vi "Camera.vi"(11 "error in (no error)":errorcluster) -> (0 "Time Out (ms) 2":u8, 1 "Camera 2":bool, 2 "Feature listout":u16, 3 "Out":bool)   [LabVIEW 2015]
uses:
  Control Button/Exit.ctl
  Control PB/Next_.ctl
panel:
  in  "Feature list":u16(ring) items=["LCD/TFT & Dail Check Camera", "CAM2", "CAM3"]
  in  "Camera":bool
  in  "Time Out (ms)":u8
  in  "Next":T1
  in  "Exit":T2
  # "Add Feature List"
  # "CAM1"
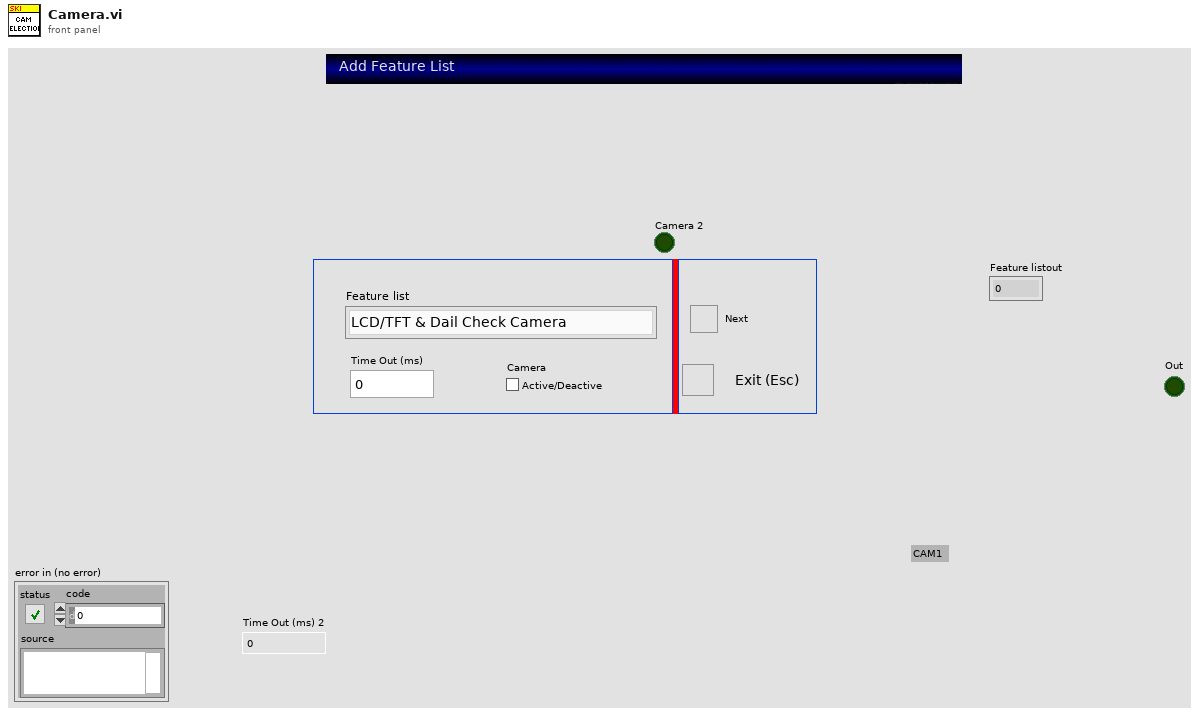
[diagram p1: front panel]
types:
  T1 = typedef "Next_.ctl" = bool
  T2 = typedef "Exit.ctl" = bool
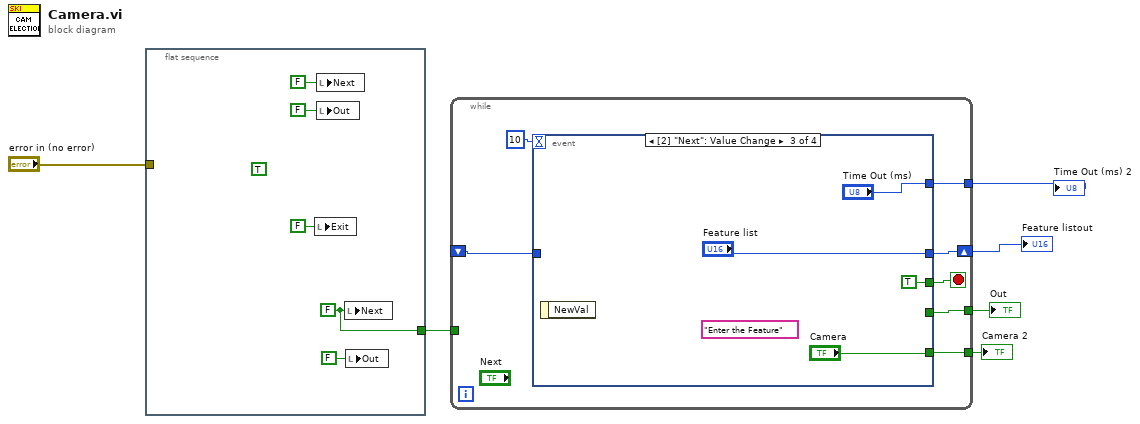
[diagram p0: block diagram]
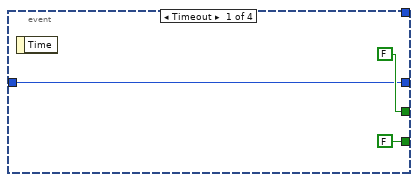
[diagram p2: hidden frame]
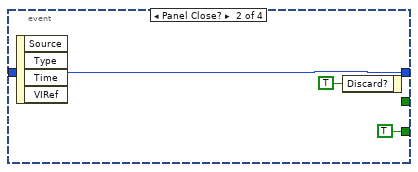
[diagram p3: hidden frame]
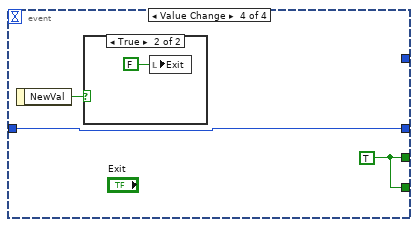
[diagram p4: hidden frame]
diagram:
  n1 = flat-sequence {
    tunnel: [w8] -> w5
    tunnel: "error in (no error)" -> [_]
    frame #0 {
      w8 = T1 FALSE ("Next")
      (unwired) TRUE ("Key Focus")
      n2 = local write "Exit"(FALSE ("Exit")) -> ()
      n3 = local write "Next"(T1 FALSE ("Next")) -> ()
      n4 = local write "Out"(FALSE ("Out")) -> ()
      n5 = local write "Next"(w8) -> ()
      n6 = local write "Out"(FALSE ("Out")) -> ()
    }
  }
  n7 = while {
    tunnel: [w16] -> w6
    tunnel: w5 -> [_]
    shift-right: [w17] -> w1
    shift-left: _ -> [w14]
    tunnel: [w13] -> w4
    tunnel: [w12] -> w3
    stop <- w18 stop-if-true
    n8 = event shown="[2] \"Next\": Value Change" {
      selector: _ -> [_ _ _ _]
      dyn-events: _ -> [_ _ _ _]
      timeout: 10 -> [_ _ _ _]
      tunnel: [FALSE _ TRUE w29] -> w18
      tunnel: [w19 w22 "Feature list" w30] -> w17
      tunnel: [T1 FALSE ("NewVal") T1 TRUE ("NewVal") _ w29] -> w16
      tunnel: w14 -> [w19 w22 _ w30]
      tunnel: [_ _ "Time Out (ms)" _] -> w13
      tunnel: [_ _ "Camera" _] -> w12
      event Timeout {
        n9 = event-data() -> ()  [unwired: 1 in, 1 out]
      }
      event Panel Close? {
        n10 = event-data() -> ()  [unwired: 1 in, 4 out]
        n11 = event-data("Discard?"=TRUE) -> ()  [unwired: 1 in, 1 out]
      }
      event Value Change {
        (unwired) "Enter the Feature"
        n12 = event-data() -> ()  [unwired: 1 in, 1 out]
      }
      event Value Change {
        w29 = TRUE
        n13 = event-data() -> ("NewVal"=w31:T2)  [unwired: 1 in]
        n14 = case shown="True" w31 {
          frame False {
          }
          frame True {
            n15 = local write "Exit"(T1 FALSE ("Next")) -> ()
          }
        }
      }
    }
  }
  "Out" <- w6
  "Time Out (ms) 2" <- w4
  "Camera 2" <- w3
  "Feature listout" <- w1
